vi "Files_ListFiles.vi"(4 "SearchOption (TopDirectory)":i32(ring) items=["TopDirectoryOnly", "AllDirectories"], 6 "SearchPattern (*)":string="*", 8 "error in (no error)":errorcluster, 11 "FolderPath In":path) -> (0 "error out":errorcluster, 1 "FilesNames":string[](array[string]), 2 "FilesPaths":path[](array[path]), 3 "FolderPath Out":path)   [LabVIEW 2021, in "LUGE_2022.4.lvlib"]
uses:
  LUGE_2022.4.lvlib
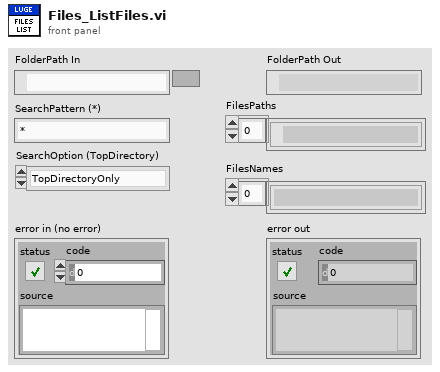
[diagram p1: front panel]
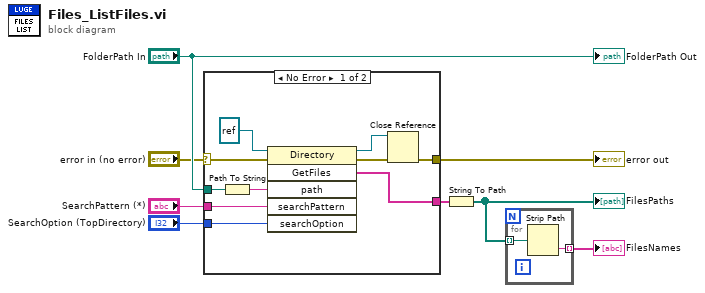
[diagram p0: block diagram]
diagram:
  n1 = case shown="No Error" "error in (no error)" {
    selector: "error in (no error)" -> [w15 w19]
    tunnel: "FolderPath In" -> [w17 _]
    tunnel: [w12 w19] -> w5
    tunnel: "SearchPattern (*)" -> [w11 _]
    tunnel: "SearchOption (TopDirectory)" -> [w10 _]
    tunnel: [w9 _] -> w4
    frame No Error {
      n2 = Path To String(path=w17) -> (string=w16:string)
      n3 = invoke class="Directory" method="GetFiles"(reference=refnum<k24> refnum, error in=w15, "path"=w16, "searchPattern"=w11, "searchOption"=w10) -> (reference out=w14:refnum<k24>, error out=w13:errorcluster, "GetFiles"=w9:string[])  [unwired: 1 in, 3 out]
      n4 = Close Reference(reference=w14, error in (no error)=w13) -> (error out=w12:errorcluster)
    }
    frame Error {
    }
  }
  "error out" <- w5
  n5 = String To Path(string=w4) -> (path=w2:path[])
  "FilesPaths" <- w2
  n6 = for {
    tunnel: w2 -> [w21] mode=indexing
    tunnel: [w20] -> w1 mode=indexing
    n7 = Strip Path(path=w21) -> (name=w20:string)  [unwired: 1 out]
  }
  "FilesNames" <- w1
  "FolderPath Out" <- "FolderPath In"
